vi "APC_Pcyl_Diag.vi"(2 "Expected IMEP":dbl=5.0, 3 "CombustionAnalysisCluster":T1={"IMEPn [bar]"=[nan, nan, nan, nan, nan, nan], "IMEPg [bar]"=[nan, nan, nan, nan, nan, nan], "MAPO [bar/CAD]"=[nan, nan, nan, nan, nan, nan], "maxQ [J]"=[nan, nan, nan, nan, nan, nan], "CA10  [CADATDC]"=[nan, nan, nan, nan, nan, nan], "CA50 [CADATDC]"=[nan, nan, nan, nan, nan, nan], "CA90 [CADATDC]"=[nan, nan, nan, nan, nan, nan], "Pmax [bar]"=[nan, nan, nan, nan, nan, nan], "IMEPstd [bar]"=[nan, nan, nan, nan, nan, nan], "CA03  [CADATDC]"=[nan, nan, nan, nan, nan, nan], "CA97  [CADATDC]"=[nan, nan, nan, nan, nan, nan], "CA10CA90 [CADATDC]"=[nan, nan, nan, nan, nan, nan], "maxdpdCAD [bar/CAD]"=[nan, nan, nan, nan, nan, nan], "kappa_comp [-]"=[nan, nan, nan, nan, nan, nan], "kappa_exp [-]"=[nan, nan, nan, nan, nan, nan], "PMEP [bar]"=[nan, nan, nan, nan, nan, nan], "RI [-]"=[nan, nan, nan, nan, nan, nan]}) -> (0 "WarningsAndErrors":T2[](array[typedef]), 1 "CombustionAnalysisClusterOut":T1={"IMEPn [bar]"=[nan, nan, nan, nan, nan, nan], "IMEPg [bar]"=[nan, nan, nan, nan, nan, nan], "MAPO [bar/CAD]"=[nan, nan, nan, nan, nan, nan], "maxQ [J]"=[nan, nan, nan, nan, nan, nan], "CA10  [CADATDC]"=[nan, nan, nan, nan, nan, nan], "CA50 [CADATDC]"=[nan, nan, nan, nan, nan, nan], "CA90 [CADATDC]"=[nan, nan, nan, nan, nan, nan], "Pmax [bar]"=[nan, nan, nan, nan, nan, nan], "IMEPstd [bar]"=[nan, nan, nan, nan, nan, nan], "CA03  [CADATDC]"=[nan, nan, nan, nan, nan, nan], "CA97  [CADATDC]"=[nan, nan, nan, nan, nan, nan], "CA10CA90 [CADATDC]"=[nan, nan, nan, nan, nan, nan], "maxdpdCAD [bar/CAD]"=[nan, nan, nan, nan, nan, nan], "kappa_comp [-]"=[nan, nan, nan, nan, nan, nan], "kappa_exp [-]"=[nan, nan, nan, nan, nan, nan], "PMEP [bar]"=[nan, nan, nan, nan, nan, nan], "RI [-]"=[nan, nan, nan, nan, nan, nan]})   [LabVIEW 2020]
uses:
  controls/APC_CombustionMetrics.ctl
  controls/APC_PcylDiag.ctl
  controls/APC_CylDaignosticsCluster.ctl
  <vilib>/Analysis/baseanly.llb/Mean (DBL).vi
  <vilib>/ptbypt/NI_PtbyPt.lvlib
  <vilib>/Analysis/NI_AALBase.lvlib
panel:
  in  "Load INI on startup":bool=TRUE
  in  "CA50maxError [CADATDC]":dbl=15.0
  in  "MAPOmaxError [bar/CAD]":dbl=1.0
  in  "MaxDevFromExpectedIMEPError [bar]":dbl=2.0
  in  "MaxDevFromSelfAvgError [bar]":dbl=2.0
  in  "MaxDevFromAvgError [bar]":dbl=2.0
  in  "MaxIMEPstdError [bar]":dbl=0.5
  in  "MaxPCylMaxError [bar]":dbl=1000.0
  in  "samples for running IMEP std":i32=100
  in  "CA50maxWarning [CADATDC]":dbl=15.0
  in  "MaxDevFromExpectedIMEPWarning [bar]":dbl=2.0
  in  "MaxPCylMaxWarning [bar]":dbl=100.0
  in  "MaxIMEPstdWarning [bar]":dbl=0.5
  in  "MaxDevFromSelfAvgWarning [bar]":dbl=2.0
  in  "MaxDevFromAvgWarning [bar]":dbl=2.0
  in  "MAPOmaxWarning [bar/CAD]":dbl=1.0
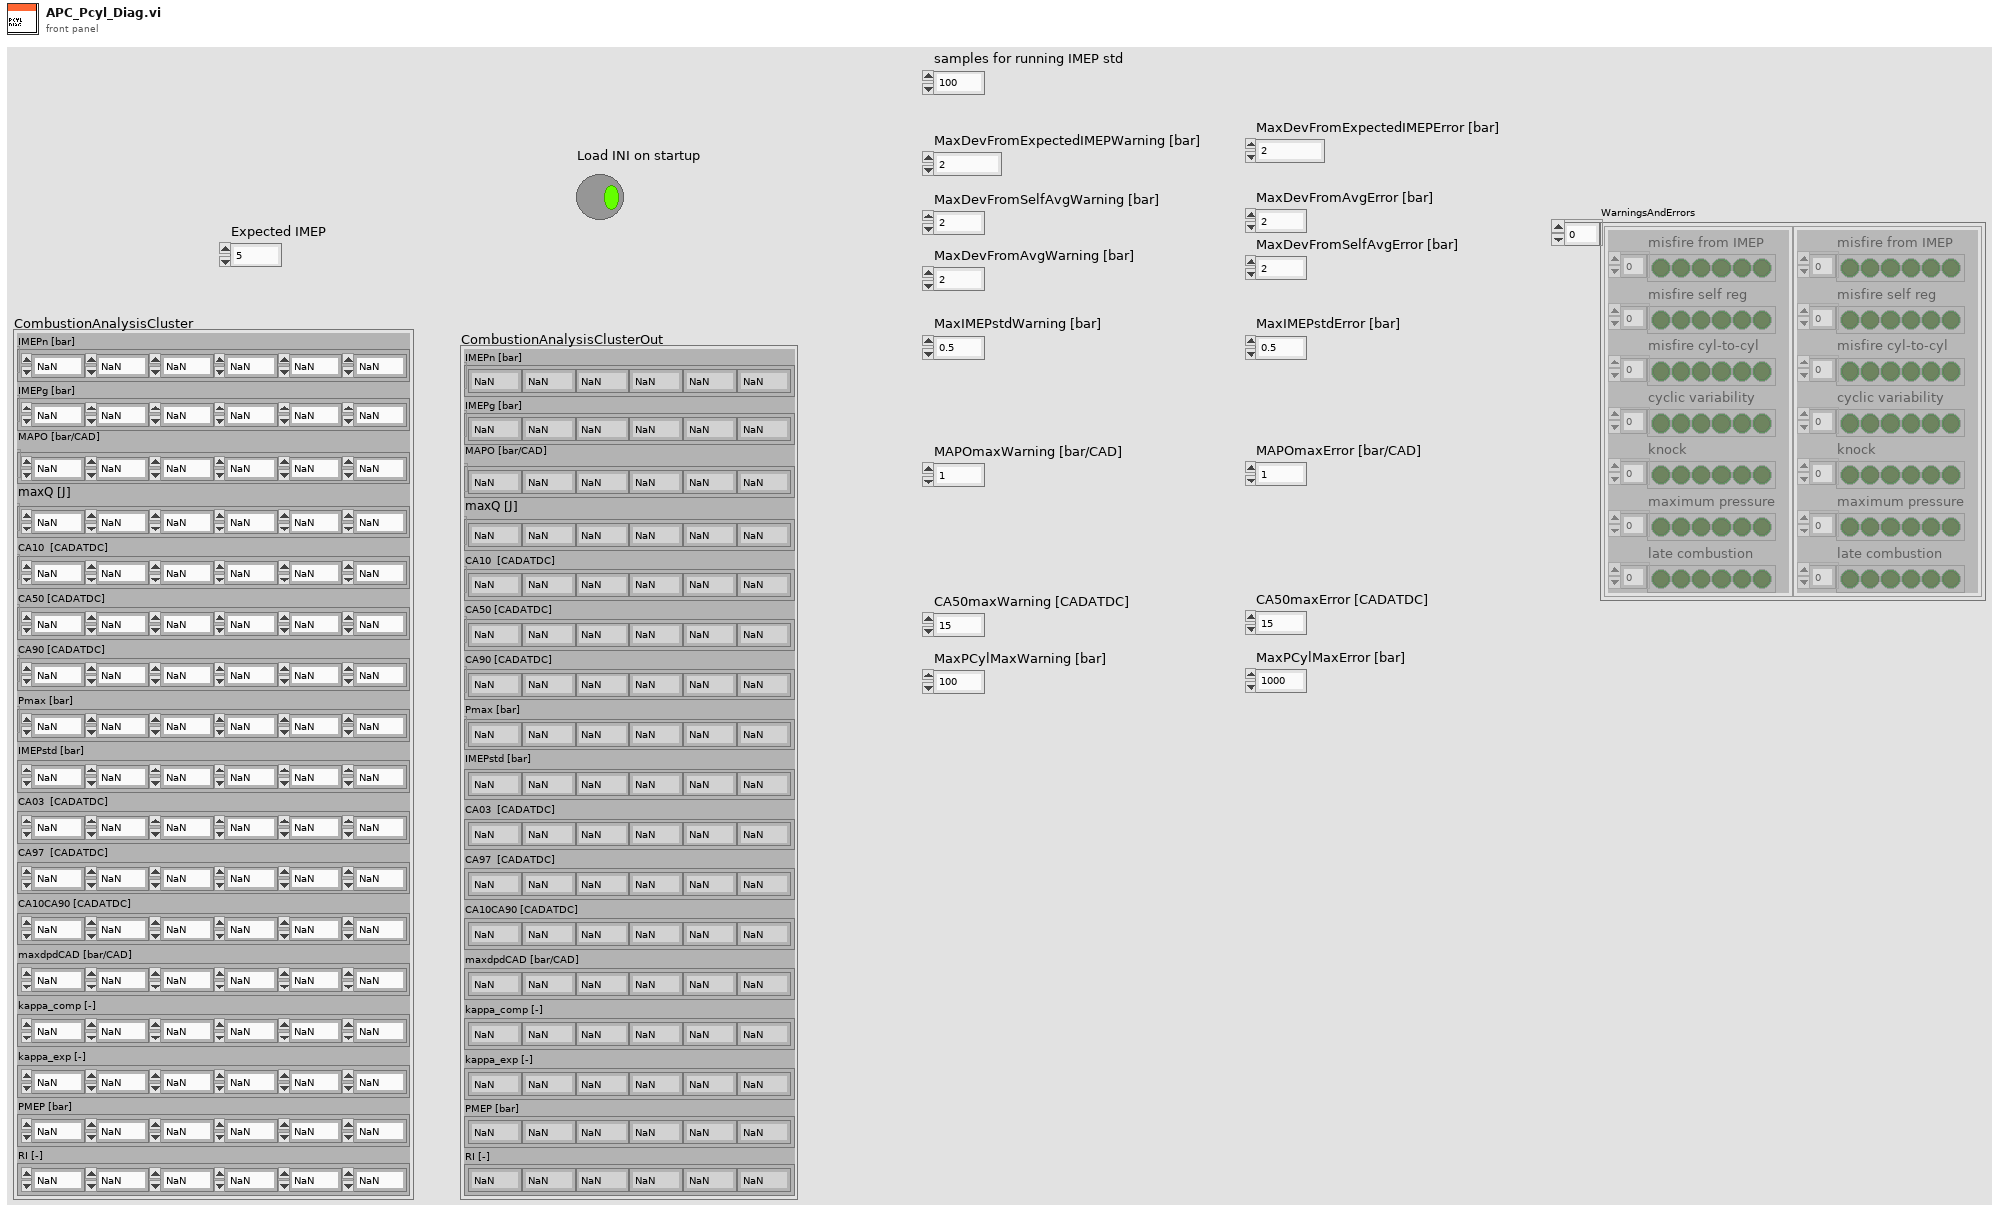
[diagram p1: front panel]
types:
  T1 = typedef "APC_CombustionMetrics.ctl" = cluster{"IMEPn [bar]":dbl[], "IMEPg [bar]":dbl[], "MAPO [bar/CAD]":dbl[], "maxQ [J]":dbl[], "CA10  [CADATDC]":dbl[], "CA50 [CADATDC]":dbl[], "CA90 [CADATDC]":dbl[], "Pmax [bar]":dbl[], "IMEPstd [bar]":dbl[], "CA03  [CADATDC]":dbl[], "CA97  [CADATDC]":dbl[], "CA10CA90 [CADATDC]":dbl[], "maxdpdCAD [bar/CAD]":dbl[], "kappa_comp [-]":dbl[], "kappa_exp [-]":dbl[], "PMEP [bar]":dbl[], "RI [-]":dbl[]}
  T2 = typedef "APC_PcylDiag.ctl" = cluster{"misfire from IMEP":bool[], "misfire self reg":bool[], "misfire cyl-to-cyl":bool[], "cyclic variability":bool[], "knock":bool[], "maximum pressure":bool[], "late combustion":bool[]}
  T3 = typedef "APC_CylDaignosticsCluster.ctl" = cluster{"samples for running IMEP std":i32, "MaxDevFromExpectedIMEPError [bar]":dbl, "MaxDevFromExpectedIMEPWarning [bar]":dbl, "MaxDevFromAvgError [bar]":dbl, "MaxDevFromSelfAvgWarning [bar]":dbl, "MaxDevFromSelfAvgError [bar]":dbl, "MaxDevFromAvgWarning [bar]":dbl, "MaxIMEPstdWarning [bar]":dbl, "MaxIMEPstdError [bar]":dbl, "MAPOmaxError [bar/CAD]":dbl, "MAPOmaxWarning [bar/CAD]":dbl, "CA50maxError [CADATDC]":dbl, "CA50maxWarning [CADATDC]":dbl, "MaxPCylMaxError [bar]":dbl, "MaxPCylMaxWarning [bar]":dbl}
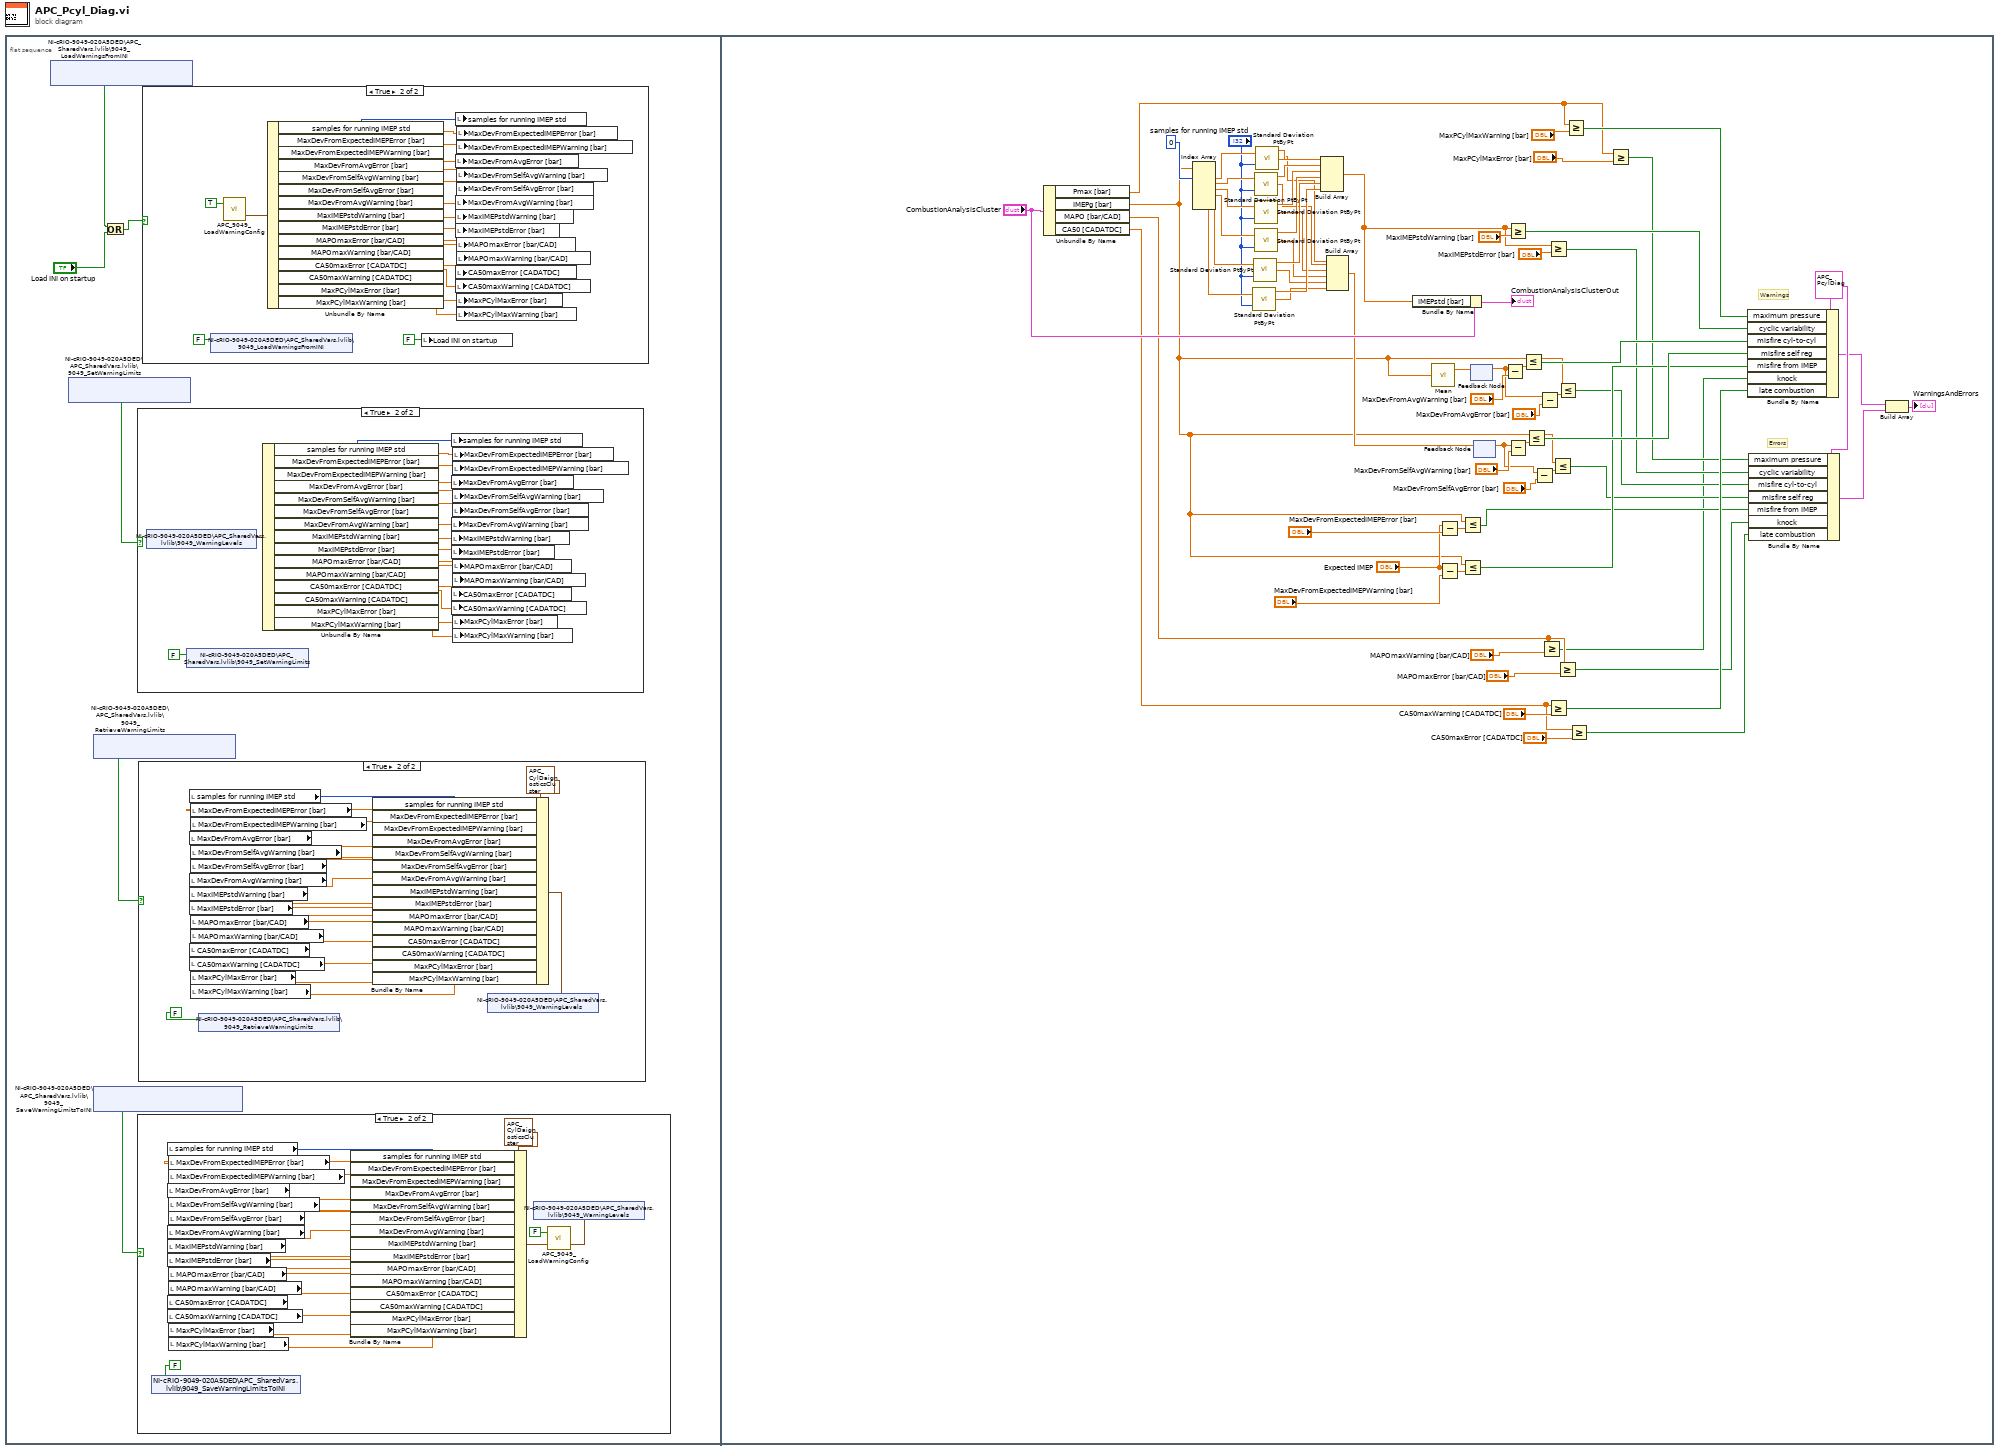
[diagram p0: block diagram]
diagram:
  n1 = flat-sequence {
    frame #0 {
      n2 = shared-variable "NI-cRIO-9049-020A5DED\\APC_SharedVars.lvlib\\9049_LoadWarningsFromINI"() -> (w3:bool)  [unwired: 1 in, 2 out]
      n3 = shared-variable "NI-cRIO-9049-020A5DED\\APC_SharedVars.lvlib\\9049_SetWarningLimits"() -> (w6:bool)  [unwired: 2 in, 2 out]
      n4 = shared-variable "NI-cRIO-9049-020A5DED\\APC_SharedVars.lvlib\\9049_SaveWarningLimitsToINI"() -> (w4:bool)  [unwired: 2 in, 2 out]
      n5 = shared-variable "NI-cRIO-9049-020A5DED\\APC_SharedVars.lvlib\\9049_RetrieveWarningLimits"() -> (w5:bool)  [unwired: 2 in, 2 out]
      n6 = Or(x=w3, y="Load INI on startup") -> (x .or. y?=w1:bool)
      n7 = case shown="True" w6 {
        frame False {
        }
        frame True {
          n8 = shared-variable "NI-cRIO-9049-020A5DED\\APC_SharedVars.lvlib\\9049_WarningLevels"() -> (w46:T3)  [unwired: 1 in, 1 out]
          n9 = shared-variable "NI-cRIO-9049-020A5DED\\APC_SharedVars.lvlib\\9049_SetWarningLimits"(FALSE ("9056SetWarningLimits")) -> ()  [unwired: 1 in, 1 out]
          n10 = Unbundle By Name(w46) -> ("samples for running IMEP std"=w61:i32, "MaxDevFromExpectedIMEPError [bar]"=w47:dbl, "MaxDevFromExpectedIMEPWarning [bar]"=w48:dbl, "MaxDevFromAvgError [bar]"=w49:dbl, "MaxDevFromSelfAvgWarning [bar]"=w50:dbl, "MaxDevFromSelfAvgError [bar]"=w51:dbl, "MaxDevFromAvgWarning [bar]"=w52:dbl, "MaxIMEPstdWarning [bar]"=w53:dbl, "MaxIMEPstdError [bar]"=w54:dbl, "MAPOmaxError [bar/CAD]"=w55:dbl, "MAPOmaxWarning [bar/CAD]"=w56:dbl, "CA50maxError [CADATDC]"=w57:dbl, "CA50maxWarning [CADATDC]"=w58:dbl, "MaxPCylMaxError [bar]"=w59:dbl, "MaxPCylMaxWarning [bar]"=w60:dbl)
          n11 = local write "samples for running IMEP std"(w61) -> ()
          n12 = local write "MaxDevFromAvgError [bar]"(w49) -> ()
          n13 = local write "MaxDevFromAvgWarning [bar]"(w52) -> ()
          n14 = local write "MaxIMEPstdWarning [bar]"(w53) -> ()
          n15 = local write "MaxIMEPstdError [bar]"(w54) -> ()
          n16 = local write "CA50maxError [CADATDC]"(w57) -> ()
          n17 = local write "CA50maxWarning [CADATDC]"(w58) -> ()
          n18 = local write "MaxDevFromExpectedIMEPError [bar]"(w47) -> ()
          n19 = local write "MaxDevFromExpectedIMEPWarning [bar]"(w48) -> ()
          n20 = local write "MaxDevFromSelfAvgWarning [bar]"(w50) -> ()
          n21 = local write "MaxDevFromSelfAvgError [bar]"(w51) -> ()
          n22 = local write "MAPOmaxError [bar/CAD]"(w55) -> ()
          n23 = local write "MAPOmaxWarning [bar/CAD]"(w56) -> ()
          n24 = local write "MaxPCylMaxError [bar]"(w59) -> ()
          n25 = local write "MaxPCylMaxWarning [bar]"(w60) -> ()
        }
      }
      n26 = case shown="True" w4 {
        frame False {
        }
        frame True {
          n27 = shared-variable "NI-cRIO-9049-020A5DED\\APC_SharedVars.lvlib\\9049_SaveWarningLimitsToINI"(FALSE ("9056SetWarningLimits")) -> ()  [unwired: 1 in, 1 out]
          n28 = local read "samples for running IMEP std"() -> (w26:i32)
          n29 = local read "MaxDevFromAvgError [bar]"() -> (w14:dbl)
          n30 = local read "MaxDevFromAvgWarning [bar]"() -> (w17:dbl)
          n31 = local read "MaxIMEPstdWarning [bar]"() -> (w18:dbl)
          n32 = local read "MaxIMEPstdError [bar]"() -> (w19:dbl)
          n33 = local read "CA50maxError [CADATDC]"() -> (w22:dbl)
          n34 = local read "CA50maxWarning [CADATDC]"() -> (w23:dbl)
          n35 = local read "MaxDevFromExpectedIMEPError [bar]"() -> (w12:dbl)
          n36 = local read "MaxDevFromExpectedIMEPWarning [bar]"() -> (w13:dbl)
          n37 = local read "MaxDevFromSelfAvgWarning [bar]"() -> (w15:dbl)
          n38 = local read "MaxDevFromSelfAvgError [bar]"() -> (w16:dbl)
          n39 = local read "MAPOmaxError [bar/CAD]"() -> (w20:dbl)
          n40 = local read "MAPOmaxWarning [bar/CAD]"() -> (w21:dbl)
          n41 = local read "MaxPCylMaxError [bar]"() -> (w24:dbl)
          n42 = local read "MaxPCylMaxWarning [bar]"() -> (w25:dbl)
          n43 = Bundle By Name(cluster=T3 {"samples for running IMEP std"=100, "MaxDevFromExpectedIMEPError [bar]"=2.0, "MaxDevFromExpectedIMEPWarning [bar]"=2.0, "MaxDevFromAvgError [bar]"=2.0, "MaxDevFromSelfAvgWarning [bar]"=2.0, "MaxDevFromSelfAvgError [bar]"=2.0, "MaxDevFromAvgWarning [bar]"=2.0, "MaxIMEPstdWarning [bar]"=0.5, "MaxIMEPstdError [bar]"=0.5, "MAPOmaxError [bar/CAD]"=1.0, "MAPOmaxWarning [bar/CAD]"=1.0, "CA50maxError [CADATDC]"=15.0, "CA50maxWarning [CADATDC]"=15.0, "MaxPCylMaxError [bar]"=120.0, "MaxPCylMaxWarning [bar]"=120.0} ("9049_WarningLevels"), "samples for running IMEP std"=w26, "MaxDevFromExpectedIMEPError [bar]"=w12, "MaxDevFromExpectedIMEPWarning [bar]"=w13, "MaxDevFromAvgError [bar]"=w14, "MaxDevFromSelfAvgWarning [bar]"=w15, "MaxDevFromSelfAvgError [bar]"=w16, "MaxDevFromAvgWarning [bar]"=w17, "MaxIMEPstdWarning [bar]"=w18, "MaxIMEPstdError [bar]"=w19, "MAPOmaxError [bar/CAD]"=w20, "MAPOmaxWarning [bar/CAD]"=w21, "CA50maxError [CADATDC]"=w22, "CA50maxWarning [CADATDC]"=w23, "MaxPCylMaxError [bar]"=w24, "MaxPCylMaxWarning [bar]"=w25) -> (w8:T3)
          n44 = call "APC_9049_LoadWarningConfig.vi"("CylinderDiagnosticsCluster"=w8, "Load?"=FALSE) -> ("CylinderDiagnosticsCluster 2"=w7:T3)  [unwired: 1 in]
          n45 = shared-variable "NI-cRIO-9049-020A5DED\\APC_SharedVars.lvlib\\9049_WarningLevels"(w7) -> ()  [unwired: 1 in, 1 out]
        }
      }
      n46 = case shown="True" w5 {
        frame False {
        }
        frame True {
          n47 = local read "samples for running IMEP std"() -> (w44:i32)
          n48 = local read "MaxDevFromAvgError [bar]"() -> (w32:dbl)
          n49 = local read "MaxDevFromAvgWarning [bar]"() -> (w35:dbl)
          n50 = local read "MaxIMEPstdWarning [bar]"() -> (w36:dbl)
          n51 = local read "MaxIMEPstdError [bar]"() -> (w37:dbl)
          n52 = local read "CA50maxError [CADATDC]"() -> (w40:dbl)
          n53 = local read "CA50maxWarning [CADATDC]"() -> (w41:dbl)
          n54 = local read "MaxDevFromExpectedIMEPError [bar]"() -> (w30:dbl)
          n55 = local read "MaxDevFromExpectedIMEPWarning [bar]"() -> (w31:dbl)
          n56 = local read "MaxDevFromSelfAvgWarning [bar]"() -> (w33:dbl)
          n57 = local read "MaxDevFromSelfAvgError [bar]"() -> (w34:dbl)
          n58 = local read "MAPOmaxError [bar/CAD]"() -> (w38:dbl)
          n59 = local read "MAPOmaxWarning [bar/CAD]"() -> (w39:dbl)
          n60 = local read "MaxPCylMaxError [bar]"() -> (w42:dbl)
          n61 = local read "MaxPCylMaxWarning [bar]"() -> (w43:dbl)
          n62 = shared-variable "NI-cRIO-9049-020A5DED\\APC_SharedVars.lvlib\\9049_RetrieveWarningLimits"(FALSE ("9056SetWarningLimits")) -> ()  [unwired: 1 in, 1 out]
          n63 = Bundle By Name(cluster=T3 {"samples for running IMEP std"=100, "MaxDevFromExpectedIMEPError [bar]"=2.0, "MaxDevFromExpectedIMEPWarning [bar]"=2.0, "MaxDevFromAvgError [bar]"=2.0, "MaxDevFromSelfAvgWarning [bar]"=2.0, "MaxDevFromSelfAvgError [bar]"=2.0, "MaxDevFromAvgWarning [bar]"=2.0, "MaxIMEPstdWarning [bar]"=0.5, "MaxIMEPstdError [bar]"=0.5, "MAPOmaxError [bar/CAD]"=1.0, "MAPOmaxWarning [bar/CAD]"=1.0, "CA50maxError [CADATDC]"=15.0, "CA50maxWarning [CADATDC]"=15.0, "MaxPCylMaxError [bar]"=120.0, "MaxPCylMaxWarning [bar]"=120.0} ("9049_WarningLevels"), "samples for running IMEP std"=w44, "MaxDevFromExpectedIMEPError [bar]"=w30, "MaxDevFromExpectedIMEPWarning [bar]"=w31, "MaxDevFromAvgError [bar]"=w32, "MaxDevFromSelfAvgWarning [bar]"=w33, "MaxDevFromSelfAvgError [bar]"=w34, "MaxDevFromAvgWarning [bar]"=w35, "MaxIMEPstdWarning [bar]"=w36, "MaxIMEPstdError [bar]"=w37, "MAPOmaxError [bar/CAD]"=w38, "MAPOmaxWarning [bar/CAD]"=w39, "CA50maxError [CADATDC]"=w40, "CA50maxWarning [CADATDC]"=w41, "MaxPCylMaxError [bar]"=w42, "MaxPCylMaxWarning [bar]"=w43) -> (w28:T3)
          n64 = shared-variable "NI-cRIO-9049-020A5DED\\APC_SharedVars.lvlib\\9049_WarningLevels"(w28) -> ()  [unwired: 1 in, 1 out]
        }
      }
      n65 = case shown="True" w1 {
        frame False {
        }
        frame True {
          n66 = shared-variable "NI-cRIO-9049-020A5DED\\APC_SharedVars.lvlib\\9049_LoadWarningsFromINI"(FALSE ("9049LoadWarningsFromINI")) -> ()  [unwired: 1 in, 1 out]
          n67 = call "APC_9049_LoadWarningConfig.vi"("Load?"=TRUE) -> ("CylinderDiagnosticsCluster 2"=w64:T3)  [unwired: 2 in]
          n68 = Unbundle By Name(w64) -> ("samples for running IMEP std"=w80:i32, "MaxDevFromExpectedIMEPError [bar]"=w66:dbl, "MaxDevFromExpectedIMEPWarning [bar]"=w67:dbl, "MaxDevFromAvgError [bar]"=w68:dbl, "MaxDevFromSelfAvgWarning [bar]"=w69:dbl, "MaxDevFromSelfAvgError [bar]"=w70:dbl, "MaxDevFromAvgWarning [bar]"=w71:dbl, "MaxIMEPstdWarning [bar]"=w72:dbl, "MaxIMEPstdError [bar]"=w73:dbl, "MAPOmaxError [bar/CAD]"=w74:dbl, "MAPOmaxWarning [bar/CAD]"=w75:dbl, "CA50maxError [CADATDC]"=w76:dbl, "CA50maxWarning [CADATDC]"=w77:dbl, "MaxPCylMaxError [bar]"=w78:dbl, "MaxPCylMaxWarning [bar]"=w79:dbl)
          n69 = local write "Load INI on startup"(FALSE ("Load INI on startup")) -> ()
          n70 = local write "samples for running IMEP std"(w80) -> ()
          n71 = local write "MaxDevFromAvgError [bar]"(w68) -> ()
          n72 = local write "MaxDevFromAvgWarning [bar]"(w71) -> ()
          n73 = local write "MaxIMEPstdWarning [bar]"(w72) -> ()
          n74 = local write "MaxIMEPstdError [bar]"(w73) -> ()
          n75 = local write "CA50maxError [CADATDC]"(w76) -> ()
          n76 = local write "CA50maxWarning [CADATDC]"(w77) -> ()
          n77 = local write "MaxDevFromExpectedIMEPError [bar]"(w66) -> ()
          n78 = local write "MaxDevFromExpectedIMEPWarning [bar]"(w67) -> ()
          n79 = local write "MaxDevFromSelfAvgWarning [bar]"(w69) -> ()
          n80 = local write "MaxDevFromSelfAvgError [bar]"(w70) -> ()
          n81 = local write "MAPOmaxError [bar/CAD]"(w74) -> ()
          n82 = local write "MAPOmaxWarning [bar/CAD]"(w75) -> ()
          n83 = local write "MaxPCylMaxError [bar]"(w78) -> ()
          n84 = local write "MaxPCylMaxWarning [bar]"(w79) -> ()
        }
      }
    }
    frame #1 {
      w85 = T2 {"misfire from IMEP"=[FALSE, FALSE, FALSE, FALSE, FALSE, FALSE], "misfire self reg"=[FALSE, FALSE, FALSE, FALSE, FALSE, FALSE], "misfire cyl-to-cyl"=[FALSE, FALSE, FALSE, FALSE, FALSE, FALSE], "cyclic variability"=[FALSE, FALSE, FALSE, FALSE, FALSE, FALSE], "knock"=[FALSE, FALSE, FALSE, FALSE, FALSE, FALSE], "maximum pressure"=[FALSE, FALSE, FALSE, FALSE, FALSE, FALSE], "late combustion"=[]} ("Cluster")
      # "Errors"
      # "Warnings"
      n85 = Unbundle By Name("CombustionAnalysisCluster") -> ("Pmax [bar]"=w110:dbl[], "IMEPg [bar]"=w97:dbl[], "MAPO [bar/CAD]"=w95:dbl[], "CA50 [CADATDC]"=w93:dbl[])
      n86 = Index Array(array=w97, index #1=0 ("index")) -> (element #1=w133:dbl, element #2=w131:dbl, element #3=w130:dbl, element #4=w129:dbl, element #5=w128:dbl, element #6=w127:dbl)  [unwired: 5 in]
      n87 = call <vilib>:"Standard Deviation PtByPt.vi"("x"=w127, "sample length"="samples for running IMEP std") -> ("standard deviation"=w120:dbl, "mean"=w118:dbl)  [unwired: 1 in, 1 out]
      n88 = call <vilib>:"Standard Deviation PtByPt.vi"("x"=w128, "sample length"="samples for running IMEP std") -> ("standard deviation"=w123:dbl, "mean"=w119:dbl)  [unwired: 1 in, 1 out]
      n89 = call <vilib>:"Standard Deviation PtByPt.vi"("x"=w131, "sample length"="samples for running IMEP std") -> ("standard deviation"=w125:dbl, "mean"=w115:dbl)  [unwired: 1 in, 1 out]
      n90 = call <vilib>:"Standard Deviation PtByPt.vi"("x"=w130, "sample length"="samples for running IMEP std") -> ("standard deviation"=w124:dbl, "mean"=w116:dbl)  [unwired: 1 in, 1 out]
      n91 = call <vilib>:"Standard Deviation PtByPt.vi"("x"=w129, "sample length"="samples for running IMEP std") -> ("standard deviation"=w122:dbl, "mean"=w117:dbl)  [unwired: 1 in, 1 out]
      n92 = call <vilib>:"Standard Deviation PtByPt.vi"("x"=w133, "sample length"="samples for running IMEP std") -> ("standard deviation"=w126:dbl, "mean"=w114:dbl)  [unwired: 1 in, 1 out]
      n93 = Build Array(w126, w125, w124, w122, w123, w120) -> (w107:dbl[])
      n94 = Build Array(w114, w115, w116, w117, w119, w118) -> (w121:dbl[])
      n95 = Bundle By Name(cluster="CombustionAnalysisCluster", "IMEPstd [bar]"=w107) -> (→"CombustionAnalysisClusterOut":T1)
      n96 = call-poly <vilib>:"Mean.vi"("X"=w97) -> ("mean"=w149:dbl)  [unwired: 1 out]
      n97 = Subtract(x="Expected IMEP", y="MaxDevFromExpectedIMEPError [bar]") -> (x-y=w100:dbl)
      n98 = Subtract(x="Expected IMEP", y="MaxDevFromExpectedIMEPWarning [bar]") -> (x-y=w142:dbl)
      n99 = Less Or Equal?(x=w97, y=w100) -> (x <= y?=w88:bool[])
      n100 = Less Or Equal?(x=w97, y=w142) -> (x <= y?=w136:bool[])
      n101 = feedback #1() -> (w104:dbl)  [unwired: 1 in]
      n102 = feedback-in #1(w149) -> ()
      n103 = feedback #2() -> (w101:dbl[])  [unwired: 1 in]
      n104 = feedback-in #2(w121) -> ()
      n105 = Subtract(x=w104, y="MaxDevFromAvgWarning [bar]") -> (x-y=w148:dbl)
      n106 = Greater Or Equal?(x=w107, y="MaxIMEPstdWarning [bar]") -> (x >= y?=w139:bool[])
      n107 = Subtract(x=w101, y="MaxDevFromSelfAvgWarning [bar]") -> (x-y=w146:dbl[])
      n108 = Less Or Equal?(x=w97, y=w148) -> (x <= y?=w138:bool[])
      n109 = Less Or Equal?(x=w97, y=w146) -> (x <= y?=w137:bool[])
      n110 = Subtract(x=w101, y="MaxDevFromSelfAvgError [bar]") -> (x-y=w103:dbl[])
      n111 = Subtract(x=w104, y="MaxDevFromAvgError [bar]") -> (x-y=w106:dbl)
      n112 = Greater Or Equal?(x=w95, y="MAPOmaxWarning [bar/CAD]") -> (x >= y?=w81:bool[])
      n113 = Greater Or Equal?(x=w107, y="MaxIMEPstdError [bar]") -> (x >= y?=w91:bool[])
      n114 = Greater Or Equal?(x=w93, y="CA50maxWarning [CADATDC]") -> (x >= y?=w112:bool[])
      n115 = Less Or Equal?(x=w97, y=w103) -> (x <= y?=w89:bool[])
      n116 = Greater Or Equal?(x=w95, y="MAPOmaxError [bar/CAD]") -> (x >= y?=w87:bool[])
      n117 = Less Or Equal?(x=w97, y=w106) -> (x <= y?=w90:bool[])
      n118 = Greater Or Equal?(x=w110, y="MaxPCylMaxWarning [bar]") -> (x >= y?=w140:bool[])
      n119 = Greater Or Equal?(x=w93, y="CA50maxError [CADATDC]") -> (x >= y?=w86:bool[])
      n120 = Greater Or Equal?(x=w110, y="MaxPCylMaxError [bar]") -> (x >= y?=w92:bool[])
      n121 = Bundle By Name(cluster=w85, "maximum pressure"=w140, "cyclic variability"=w139, "misfire cyl-to-cyl"=w138, "misfire self reg"=w137, "misfire from IMEP"=w136, "knock"=w81, "late combustion"=w112) -> (w84:T2)
      n122 = Bundle By Name(cluster=w85, "maximum pressure"=w92, "cyclic variability"=w91, "misfire cyl-to-cyl"=w90, "misfire self reg"=w89, "misfire from IMEP"=w88, "knock"=w87, "late combustion"=w86) -> (w83:T2)
      n123 = Build Array(w84, w83) -> (→"WarningsAndErrors":T2[])
    }
  }
